vi "Read Show help.vi"(11 "SolutionBuilder in":refnum<class "SolutionBuilder.lvclass">) -> (2 "Show help?":bool, 3 "SolutionBuilder out":refnum<class "SolutionBuilder.lvclass">)   [LabVIEW 2020, in "SolutionBuilder.lvlib" / "SolutionBuilder.lvclass"]
uses:
  SolutionBuilder.lvclass
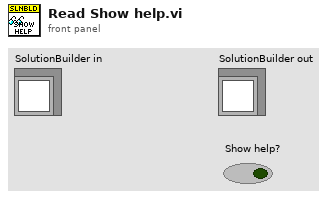
[diagram p1: front panel]
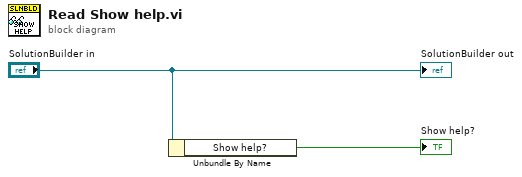
[diagram p0: block diagram]
diagram:
  n1 = Unbundle By Name("SolutionBuilder in") -> ("Show help?"=→"Show help?":bool)
  "SolutionBuilder out" <- "SolutionBuilder in"
